vi "逐点求导.vi"() -> ()   [LabVIEW 2018]
uses:
  <vilib>/ptbypt/NI_PtbyPt.lvlib
panel:
  in  "停止":bool
  out "dx/dt":dbl format="%0.2f"
  in  "x":dbl format="%0.2f"
  in  "initialize":bool caption="初始化"
  in  "dt":dbl=1.0 format="%0.2f"
  in  "initial condition":dbl caption="初始条件" format="%0.2f"
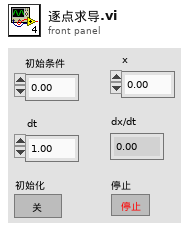
[diagram p1: front panel]
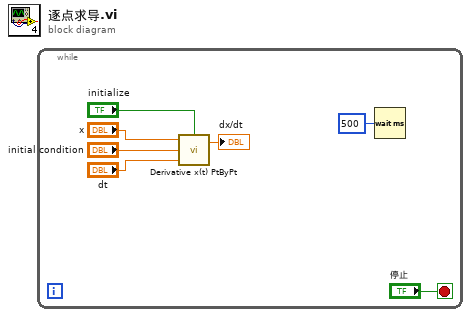
[diagram p0: block diagram]
diagram:
  n1 = while {
    stop <- "停止" stop-if-true
    n2 = call <vilib>:"Derivative x(t) PtByPt.vi"("initialize"="initialize", "dt"="dt", "initial condition"="initial condition", "x"="x") -> ("dx/dt"=→"dx/dt":dbl)  [unwired: 1 out]
    n3 = Wait (ms)(milliseconds to wait=u32 500 ("等待时间（毫秒）")) -> ()  [unwired: 1 out]
  }
